vi "unflattenMassFromXML_Array.vi"(8 "error in (no error)":errorcluster, 9 "massUnitInXML":T1, 10 "xmlString":string, 11 "massForType":dbl[unit][](array[numeric])=[0.11875020477636528, 0.23750040955273055, 0.35625061432909577, 0.4750008191054611]) -> (0 "error out":errorcluster, 3 "mass":dbl[unit][](array[numeric]))   [LabVIEW 2012, in "UnitsAndXML.lvlib"]
uses:
  <userlib>/Common/UnitsAndXML/UnitsAndXML.lvlib
  <userlib>/Common/UnitsAndXML/FlattenItemWithUnitToXML/FlattenMassToXML/MassUnit.ctl
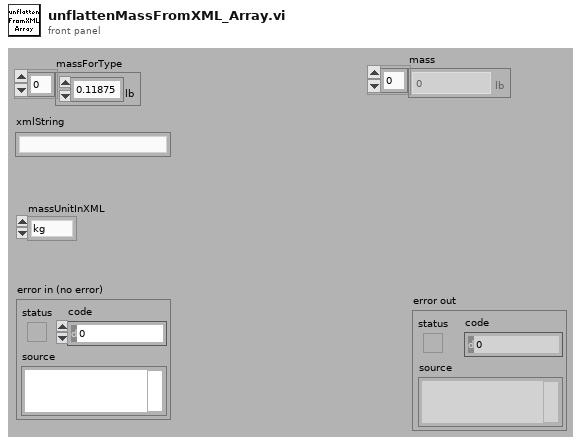
[diagram p1: front panel]
types:
  T1 = typedef "UnitsAndXML.lvlib/MassUnit.ctl" = enum16{"kg", "CM", "dr", "gr", "t", "oz", "lb", "slug", "stone", "Ton", "ton", "u"}
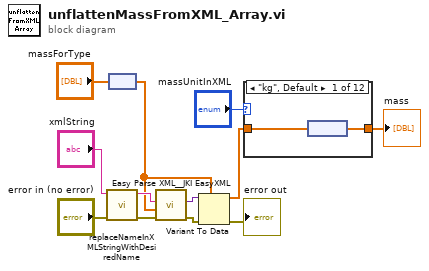
[diagram p0: block diagram]
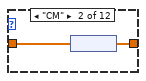
[diagram p2: hidden frame]
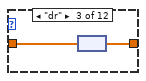
[diagram p3: hidden frame]
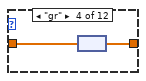
[diagram p4: hidden frame]
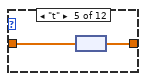
[diagram p5: hidden frame]
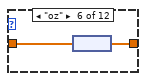
[diagram p6: hidden frame]
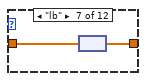
[diagram p7: hidden frame]
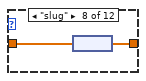
[diagram p8: hidden frame]
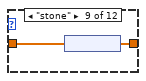
[diagram p9: hidden frame]
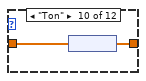
[diagram p10: hidden frame]
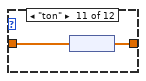
[diagram p11: hidden frame]
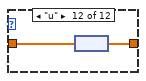
[diagram p12: hidden frame]
diagram:
  n1 = call <userlib>:"replaceNameInXMLStringWithDesiredName.vi"("error in"="error in (no error)", "xmlString"="xmlString") -> ("error out"=w5:errorcluster, "revisedXMLString"=w10:string)  [unwired: 8 in]
  n2 = node("massForType") -> (w9:dbl[])
  n3 = call <vilib>:"Easy Parse XML__JKI EasyXML.vi"("error in (no error)"=w5, "LabVIEW Data (Type)"=w9, "XML String"=w10) -> ("error out"=w8:errorcluster, "LabVIEW Data"=w12:variant)  [unwired: 7 in]
  n4 = Variant To Data(error in=w8, type=w9, Variant=w12) -> (data=w2:dbl[], error out=→"error out":errorcluster)
  n5 = case shown="\"kg\", Default" "massUnitInXML" {
    tunnel: w2 -> [w14 w16 w18 w20 w22 w24 w26 w28 w30 w32 w34 w36]
    tunnel: [w13 w15 w17 w19 w21 w23 w25 w27 w29 w31 w33 w35] -> w1
    frame "kg", Default {
      n6 = node(w14) -> (w13:dbl[unit][])
    }
    frame "CM" {
      n7 = node(w16) -> (w15:dbl[unit][])
    }
    frame "dr" {
      n8 = node(w18) -> (w17:dbl[unit][])
    }
    frame "gr" {
      n9 = node(w20) -> (w19:dbl[unit][])
    }
    frame "t" {
      n10 = node(w22) -> (w21:dbl[unit][])
    }
    frame "oz" {
      n11 = node(w24) -> (w23:dbl[unit][])
    }
    frame "lb" {
      n12 = node(w26) -> (w25:dbl[unit][])
    }
    frame "slug" {
      n13 = node(w28) -> (w27:dbl[unit][])
    }
    frame "stone" {
      n14 = node(w30) -> (w29:dbl[unit][])
    }
    frame "Ton" {
      n15 = node(w32) -> (w31:dbl[unit][])
    }
    frame "ton" {
      n16 = node(w34) -> (w33:dbl[unit][])
    }
    frame "u" {
      n17 = node(w36) -> (w35:dbl[unit][])
    }
  }
  "mass" <- w1
